vi "setSerializedData.vi"(0 "reference":refnum<class "StateNode.lvclass">, 1 "parent":refnum<class "AbstractNode.lvclass">, 2 "children":refnum<class "AbstractNode.lvclass">[](array[class]), 3 "xmlOut":string, 5 "error in (no error)":errorcluster) -> (14 "reference out":refnum<class "StateNode.lvclass">, 19 "error out":errorcluster)   [LabVIEW 2012, in "StateNode.lvclass"]
doc: "setSerializedData"
uses:
  <resource>/Framework/Providers/Open_GDS/UML/StateNode_class/StateNode.lvclass
  <resource>/Framework/Providers/Open_GDS/UML/AbstractNode_class/AbstractNode.lvclass
  <resource>/Framework/Providers/Open_GDS/UML/AbstractNode_class/ObjectReference.ctl
  <resource>/Framework/Providers/Open_GDS/UML/General/Rectangle/Rectangle Rectangle2D.ctl
  <resource>/Framework/Providers/Open_GDS/UML/MultiLineString_class/ObjectReference.ctl
  <resource>/Framework/Providers/Open_GDS/UML/MultiLineString_class/MultiLineString.lvclass
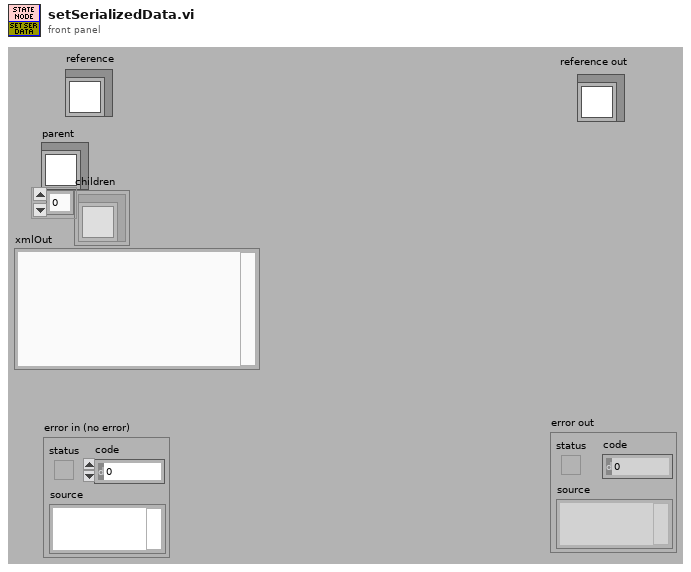
[diagram p1: front panel]
types:
  T1 = typedef "AbstractNode.lvclass/ObjectReference.ctl" = refnum<k1>
  T2 = typedef "Rectangle Rectangle2D.ctl" = cluster{"x":dbl, "y":dbl, "width":dbl, "height":dbl}
  T3 = typedef "MultiLineString.lvclass/ObjectReference.ctl" = refnum<k1>
  T4 = cluster{"Base class":cluster{"Base class":cluster{"parent":T1, "children":T1[]}, "bounds":T2}, "state":T3, "action":T3, "DEFAULT_WIDTH":i32, "DEFAULT_HEIGHT":i32}
  T5 = typedef "StateNode.lvclass/ObjectAttributes.ctl" = cluster{"Base class":T6, "state":refnum<class "MultiLineString.lvclass">, "action":refnum<class "MultiLineString.lvclass">, "DEFAULT_WIDTH":i32, "DEFAULT_HEIGHT":i32}
  T6 = typedef "RectangularNode.lvclass/ObjectAttributes.ctl" = cluster{"Base class":T7, "bounds":T2}
  T7 = typedef "AbstractNode.lvclass/ObjectAttributes.ctl" = cluster{"parent":refnum<class "AbstractNode.lvclass">, "children":refnum<class "AbstractNode.lvclass">[], "Hidden":bool}
  T8 = cluster{"Attributes":cluster{"Base class":cluster{"Base class":cluster{"parent":T1, "children":T1[]}, "bounds":T2}, "state":T3, "action":T3, "DEFAULT_WIDTH":i32, "DEFAULT_HEIGHT":i32}, string, string}
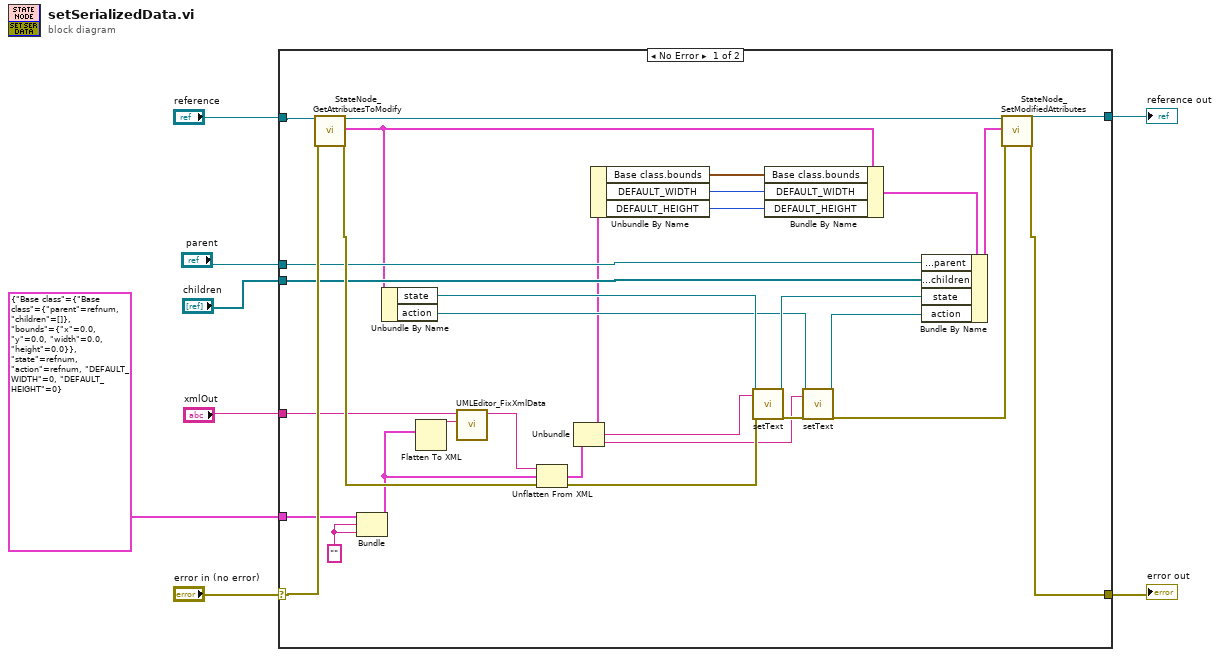
[diagram p0: block diagram]
diagram:
  n1 = case shown="No Error" "error in (no error)" {
    selector: "error in (no error)" -> [w30 w40]
    tunnel: "reference" -> [w31 w41]
    tunnel: [w29 w40] -> w6
    tunnel: [w28 w41] -> w5
    tunnel: "xmlOut" -> [w11 _]
    tunnel: "parent" -> [w27 _]
    tunnel: "children" -> [w26 _]
    tunnel: T4 {"Base class"={"Base class"={"parent"=refnum, "children"=[]}, "bounds"={"x"=0.0, "y"=0.0, "width"=0.0, "height"=0.0}}, "state"=refnum, "action"=refnum, "DEFAULT_WIDTH"=0, "DEFAULT_HEIGHT"=0} ("Attributes") -> [w19 _]
    frame No Error {
      w25 = ""
      n2 = call <resource>:"StateNode_GetAttributesToModify.vi"("reference in"=w31, "error in (no error)"=w30) -> ("reference out"=w39:refnum<class "StateNode.lvclass">, "Attributes"=w13:T5, "error out"=w37:errorcluster)  [unwired: 1 in, 14 out]
      n3 = Bundle("Attributes"=w19, w25, w25) -> (w10:T8)  [unwired: 1 out]
      n4 = Unbundle By Name(w13) -> ("state"=w36:refnum<class "MultiLineString.lvclass">, "action"=w23:refnum<class "MultiLineString.lvclass">)
      n5 = Flatten To XML(anything=w10) -> (xml string=w12:string)
      n6 = call <resource>:"UMLEditor_FixXmlData.vi"("XmlTemplateIn"=w12, "xmlIn"=w11) -> ("XML OUt"=w9:string)  [unwired: 9 in]
      n7 = Unflatten From XML(xml string=w9, type=w10, error in (no error)=w37) -> (value=w33:T8, error out=w35:errorcluster)
      n8 = Unbundle(w33) -> ("Attributes"=w15:T4, w32:string, w20:string)
      n9 = Unbundle By Name(w15) -> ("Base class.bounds"=w18:T2, "DEFAULT_WIDTH"=w17:i32, "DEFAULT_HEIGHT"=w16:i32)
      n10 = call-dynamic "setText.vi"("reference"=w36, "text"=w32, "error in (no error)"=w35) -> ("reference out"=w34:refnum<class "MultiLineString.lvclass">, "error out"=w24:errorcluster)  [unwired: 15 out]
      n11 = Bundle By Name(cluster=w13, "Base class.bounds"=w18, "DEFAULT_WIDTH"=w17, "DEFAULT_HEIGHT"=w16) -> (w14:T5)
      n12 = call-dynamic "setText.vi"("reference"=w23, "text"=w20, "error in (no error)"=w24) -> ("reference out"=w22:refnum<class "MultiLineString.lvclass">, "error out"=w21:errorcluster)  [unwired: 15 out]
      n13 = Bundle By Name(cluster=w14, "Base class.Base class.parent"=w27, "Base class.Base class.children"=w26, "state"=w34, "action"=w22) -> (w38:T5)
      n14 = call <resource>:"StateNode_SetModifiedAttributes.vi"("reference in"=w39, "Attributes"=w38, "error in (no error)"=w21) -> ("reference out"=w28:refnum<class "StateNode.lvclass">, "error out"=w29:errorcluster)  [unwired: 3 in, 12 out]
    }
    frame Error {
    }
  }
  "reference out" <- w5
  "error out" <- w6
